vi "Teleop.vi"(10 "Match Info":T1={"Autonomous Elapsed Seconds"=0.0, "TeleOp Elapsed Seconds"=0.0, "Disabled Elapsed Seconds"=0.0, "Visited Autonomous"=FALSE, "Visited TeleOp"=FALSE, "Visited Disabled"=FALSE, "Autonomous Settings"={"Autonomous Style"=enum."Independent", "VI Refnum"=refnum}}, 11 "Call Context":T2) -> ()   [LabVIEW 2017]
doc: "This VI is called for each enabled TeleOp packet received from the DS. It is typically used to read from joysticks and other inputs and update I/O or setpoints for timed control loops. It should complete and return within 20 milliseconds or risk missing DS packets."
uses:
  <vilib>/Rock Robotics/WPI/DriverStation/WPI_DriverStationDerivedRobotMode.ctl
  <vilib>/Rock Robotics/WPI/DriverStation/WPI_DriverStationMatch Info.ctl
  <vilib>/Rock Robotics/WPI/Utilities/WPI_GetSetVariantRefNum.vi
  <vilib>/Rock Robotics/Network Tables/NT Write Boolean Array.vi
  <vilib>/Rock Robotics/Network Tables/NT Write Numeric Array.vi
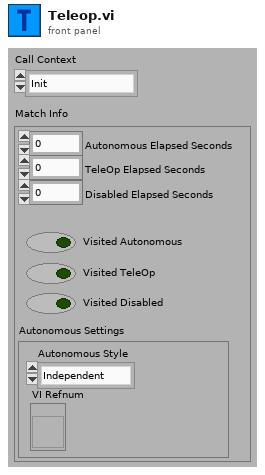
[diagram p1: front panel]
types:
  T1 = typedef "WPI_DriverStationMatch Info.ctl" = cluster{"Autonomous Elapsed Seconds":dbl, "TeleOp Elapsed Seconds":dbl, "Disabled Elapsed Seconds":dbl, "Visited Autonomous":bool, "Visited TeleOp":bool, "Visited Disabled":bool, "Autonomous Settings":cluster{"Autonomous Style":enum16{"Iterative", "Independent"}, "VI Refnum":refnum<vi>}}
  T2 = typedef "WPI_DriverStationDerivedRobotMode.ctl" = enum16{"Init", "Execute", "Stop"}
  T3 = typedef "WPI_JoystickDevRef.ctl" = cluster{"Device":T4}
  T4 = typedef "WPI_JoystickDeviceEnum.ctl" = enum16{"USB 0", "USB 1", "USB 2", "USB 3", "USB 4", "USB 5"}
  T5 = typedef "Command Status Info.ctl" = cluster{"Name":string, "Status":T6, "notifier out":T7}
  T6 = typedef "Completion Status.ctl" = enum16{"Successful", "Aborted", "Incomplete"}
  T7 = typedef "Completion Notifier.ctl" = refnum<notifier>
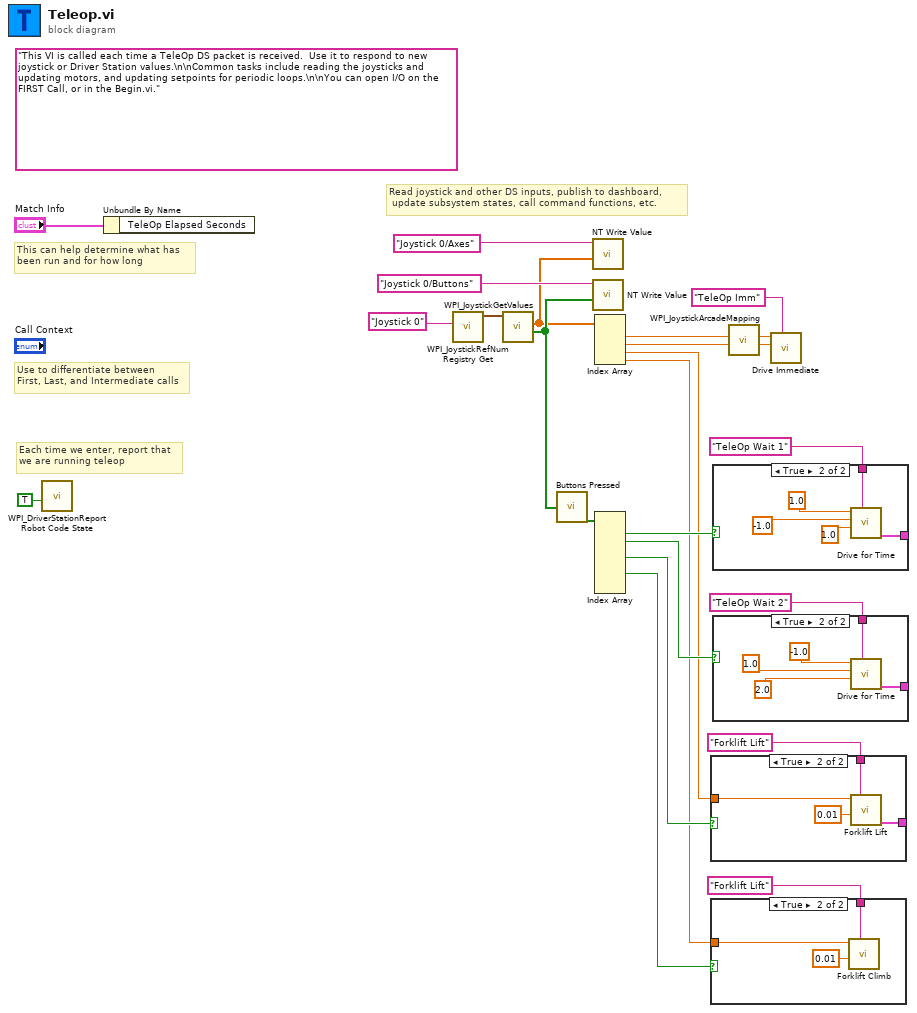
[diagram p0: block diagram]
diagram:
  (unwired) "This VI is called each time a TeleOp DS packet is received.  Use it to respond to new joystick or Driver Station values.\n\nCommon tasks include reading the joysticks and updating motors, and updating setpoints for periodic loops.\n\nYou can open I/O on the FIRST Call, or in the Begin.vi."
  # "Read joystick and other DS inputs, publish to dashboard,\n update subsystem states, call command functions, etc."
  # "Each time we enter, report that\nwe are running teleop"
  # "Use to differentiate between\nFirst, Last, and Intermediate calls"
  # "This can help determine what has\nbeen run and for how long"
  n1 = call <vilib>:"WPI_DriverStationReport Robot Code State.vi"("TeleOp"=TRUE ("Autonomous")) -> ()  [unwired: 10 in, 1 out]
  n2 = Unbundle By Name("Match Info") -> ()  [unwired: 1 out]
  n3 = call <vilib>:"WPI_JoystickRefNum Registry Get.vi"("refnum name"="Joystick 0") -> ("JoystickDevRef"=w21:T3)  [unwired: 1 in, 9 out]
  n4 = call <vilib>:"WPI_JoystickGetValues.vi"("JoystickDevRef"=w21) -> ("Buttons"=w9:bool[], "Axes"=w8:dbl[])  [unwired: 6 in, 3 out]
  n5 = call "Buttons Pressed.vi"("Button Values"=w9) -> ("Button Presses"=w17:bool[])
  n6 = call-poly <vilib>:"NT Write Value.vi"("Numeric Array"=w8, "Name"="Joystick 0/Axes") -> ()  [unwired: 9 in, 1 out]
  n7 = call-poly <vilib>:"NT Write Value.vi"("Boolean Array"=w9, "Name"="Joystick 0/Buttons") -> ()  [unwired: 9 in, 1 out]
  n8 = Index Array(array=w8) -> (element #1=w12:dbl, element #2=w11:dbl, element #3=w4:dbl, element #4=w1:dbl)  [unwired: 4 in]
  n9 = Index Array(array=w17) -> (element #1=w16:bool, element #2=w15:bool, element #4=w5:bool, element #6=w2:bool)  [unwired: 8 in, 4 out]
  n10 = case shown="True" w5 {
    tunnel: "Forklift Lift" ("Description") -> [_ w28]
    tunnel: [_ w27] -> _
    tunnel: w4 -> [_ w25]
    frame False {
    }
    frame True {
      n11 = call "Forklift Lift.vi"("Description"=w28, "Deadband Value"=0.01, "Setpoint"=w25) -> ("Command Info Out"=w27:T5)  [unwired: 8 in]
    }
  }
  n12 = case shown="True" w2 {
    tunnel: "Forklift Lift" ("Description") -> [_ w31]
    tunnel: w1 -> [_ w29]
    frame False {
    }
    frame True {
      n13 = call "Forklift Climb.vi"("Description"=w31, "Deadband Value"=0.01, "Setpoint"=w29) -> ()  [unwired: 8 in, 1 out]
    }
  }
  n14 = case shown="True" w16 {
    tunnel: [_ w35] -> _
    tunnel: "TeleOp Wait 1" ("Description") -> [_ w34]
    frame False {
    }
    frame True {
      n15 = call "Drive for Time.vi"("Description"=w34, "Seconds"=1.0, "Right Speed"=-1.0, "Left Speed"=1.0) -> ("Command Info Out"=w35:T5)  [unwired: 6 in, 1 out]
    }
  }
  n16 = case shown="True" w15 {
    tunnel: [_ w39] -> _
    tunnel: "TeleOp Wait 2" ("Description") -> [_ w38]
    frame False {
    }
    frame True {
      n17 = call "Drive for Time.vi"("Description"=w38, "Seconds"=2.0, "Right Speed"=1.0, "Left Speed"=-1.0) -> ("Command Info Out"=w39:T5)  [unwired: 6 in, 1 out]
    }
  }
  n18 = call <vilib>:"WPI_JoystickArcadeMapping.vi"("Y axis value"=w11, "X axis value"=w12) -> ("Right Motor Value"=w13:dbl, "Left Motor Value"=w14:dbl)  [unwired: 8 in]
  n19 = call "Drive Immediate.vi"("Description"="TeleOp Imm", "Right Setpoint"=w13, "Left Setpoint"=w14) -> ()  [unwired: 8 in, 1 out]
